vi "Heat Tapes.vi"() -> ()   [LabVIEW 2013]
panel:
  out "Boolean 7":bool
  out "Boolean 6":bool
  out "Boolean 5":bool
  out "Boolean 4":bool
  out "Boolean 3":bool
  out "Boolean 2":bool
  out "Boolean":bool
  in  "On 8":bool
  out "HT-301 Steam":dynamicdata(graph)
  in  "HT-301 SP":dbl
  in  "Auto 7":bool=TRUE
  in  "Set All":bool
  in  "Setpoint":dbl
  in  "Auto":bool
  in  "On":bool
  in  "HT-601 SP":dbl
  in  "Auto 6":bool
  in  "HT-621 SP":dbl
  in  "On 6":bool
  in  "Auto 5":bool
  in  "HT-620 SP":dbl
  in  "On 5":bool
  in  "Auto 4":bool
  in  "HT-611 SP":dbl
  in  "On 4":bool
  in  "Auto 3":bool
  in  "HT-610 SP":dbl
  in  "On 3":bool
  in  "Auto 2":bool
  in  "HT-602 SP":dbl
  in  "On 2":bool
  out "HT-601 - Ash Knockout":dynamicdata(graph)
  out "HT-602 - Horizontal":dynamicdata(graph)
  out "HT-610 - Filter 1":dynamicdata(graph)
  out "HT-620 - Filter 2":dynamicdata(graph)
  out "HT-611 - Between Filters":dynamicdata(graph)
  out "HT-621 - Between Filter 2 & VLS":dynamicdata(graph)
  in  "Auto 9":bool=TRUE
  # "Heat Tape Control Panel (to set all)"
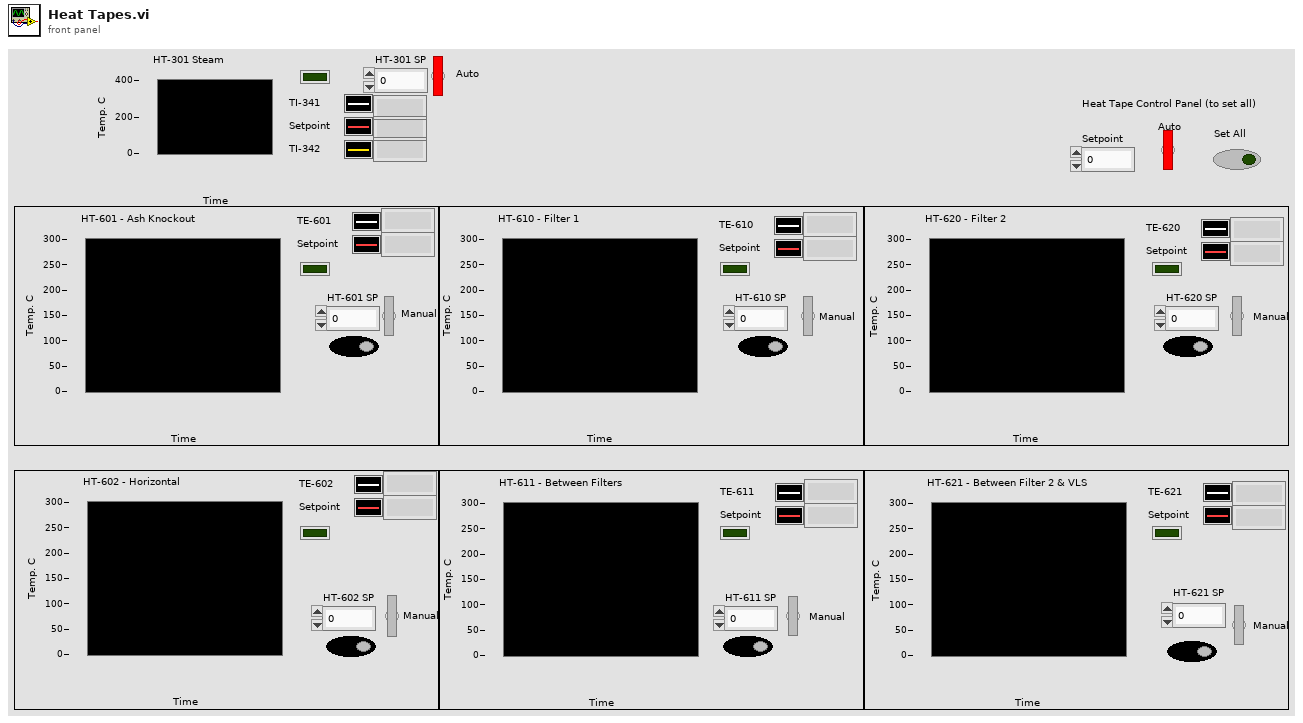
[diagram p1: front panel]
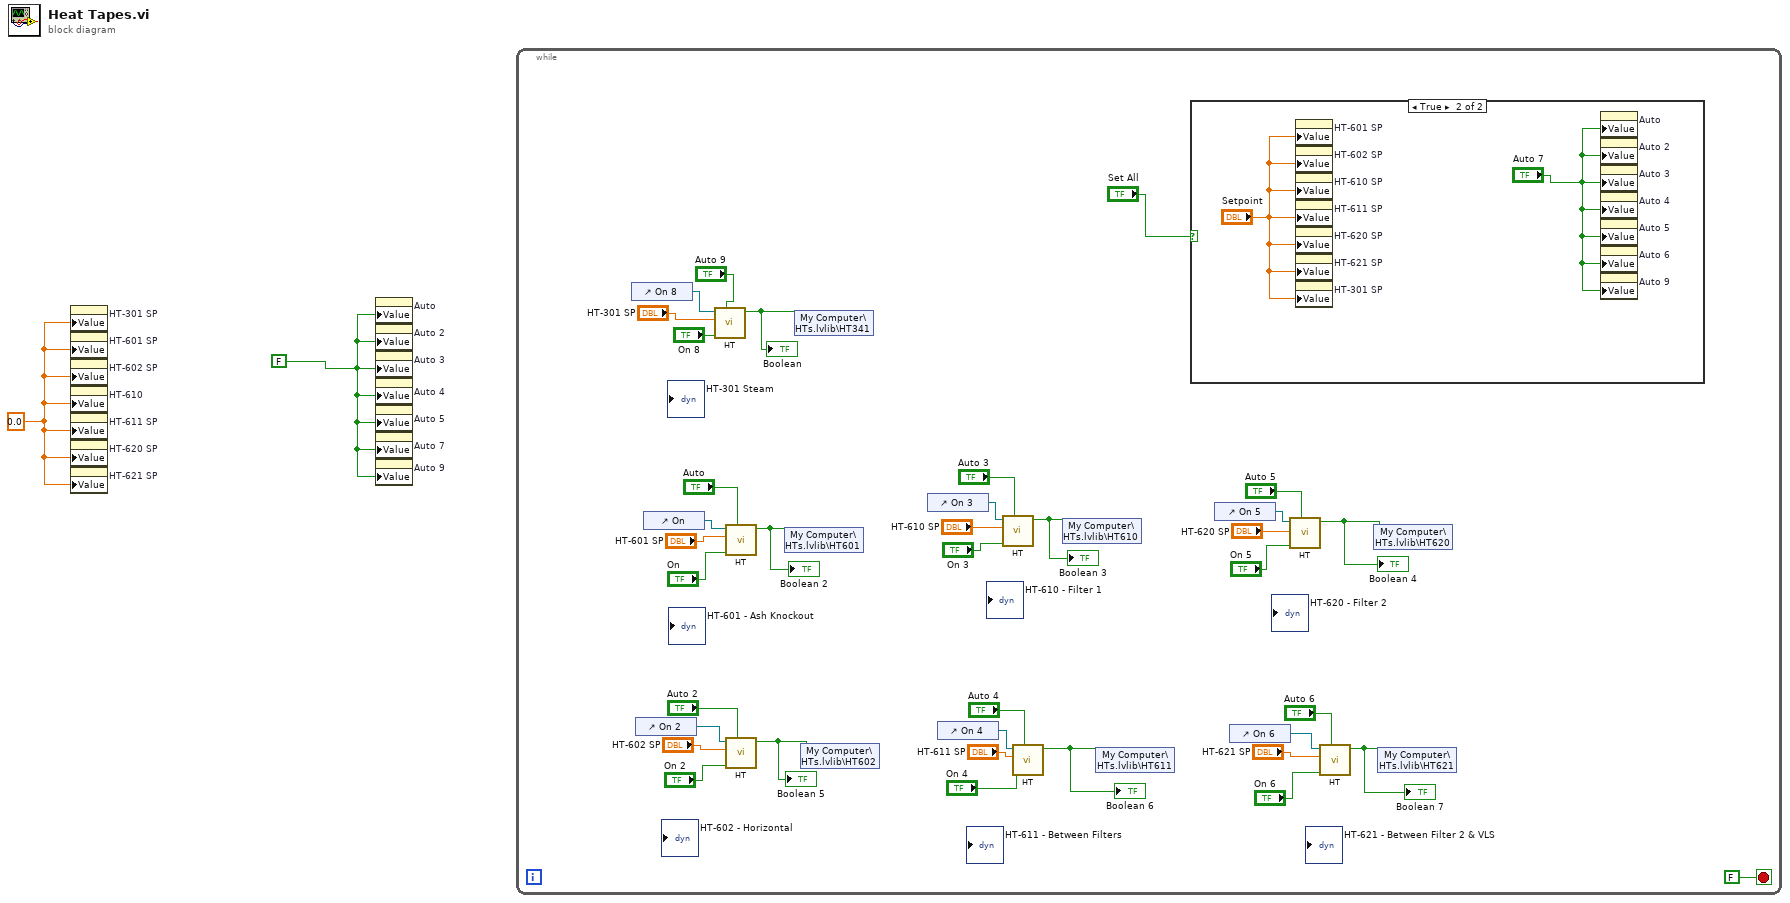
[diagram p0: block diagram]
diagram:
  w2 = FALSE ("Auto 8")
  w1 = 0.0 ("Setpoint 2")
  n1 = property on="HT-301 SP" class="DigNum (strict)"("Value"=w1) -> ()  [unwired: 2 in, 2 out]
  n2 = property on="HT-601 SP" class="DigNum (strict)"("Value"=w1) -> ()  [unwired: 2 in, 2 out]
  n3 = property on="HT-602 SP" class="DigNum (strict)"("Value"=w1) -> ()  [unwired: 2 in, 2 out]
  n4 = property on="HT-610" class="DigNum (strict)"("Value"=w1) -> ()  [unwired: 2 in, 2 out]
  n5 = property on="HT-611 SP" class="DigNum (strict)"("Value"=w1) -> ()  [unwired: 2 in, 2 out]
  n6 = property on="HT-620 SP" class="DigNum (strict)"("Value"=w1) -> ()  [unwired: 2 in, 2 out]
  n7 = property on="HT-621 SP" class="DigNum (strict)"("Value"=w1) -> ()  [unwired: 2 in, 2 out]
  n8 = property on="Auto" class="Bool (strict)"("Value"=w2) -> ()  [unwired: 2 in, 2 out]
  n9 = property on="Auto 2" class="Bool (strict)"("Value"=w2) -> ()  [unwired: 2 in, 2 out]
  n10 = property on="Auto 3" class="Bool (strict)"("Value"=w2) -> ()  [unwired: 2 in, 2 out]
  n11 = property on="Auto 4" class="Bool (strict)"("Value"=w2) -> ()  [unwired: 2 in, 2 out]
  n12 = property on="Auto 5" class="Bool (strict)"("Value"=w2) -> ()  [unwired: 2 in, 2 out]
  n13 = property on="Auto 7" class="Bool (strict)"("Value"=w2) -> ()  [unwired: 2 in, 2 out]
  n14 = property on="Auto 9" class="Bool (strict)"("Value"=w2) -> ()  [unwired: 2 in, 2 out]
  n15 = while {
    stop <- FALSE stop-if-true
    n16 = control-ref of="On 8"() -> (w12:refnum<vi>)
    n17 = control-ref of="On 2"() -> (w17:refnum<vi>)
    n18 = control-ref of="On"() -> (w16:refnum<vi>)
    n19 = call "HT.vi"("Auto"="Auto 9", "On"="On 8", "SP"="HT-301 SP", "Bool Refnum"=w12) -> ("s? t:f"=w11:bool)  [unwired: 7 in]
    "Boolean" <- w11
    n20 = call "HT.vi"("Auto"="Auto", "On"="On", "SP"="HT-601 SP", "Bool Refnum"=w16) -> ("s? t:f"=w9:bool)  [unwired: 7 in]
    "Boolean 2" <- w9
    n21 = call "HT.vi"("Auto"="Auto 2", "On"="On 2", "SP"="HT-602 SP", "Bool Refnum"=w17) -> ("s? t:f"=w6:bool)  [unwired: 7 in]
    "Boolean 5" <- w6
    n22 = shared-variable "My Computer\\HTs.lvlib\\HT601"(w9) -> ()  [unwired: 1 in, 1 out]
    n23 = shared-variable "My Computer\\HTs.lvlib\\HT341"(w11) -> ()  [unwired: 1 in, 1 out]
    n24 = shared-variable "My Computer\\HTs.lvlib\\HT602"(w6) -> ()  [unwired: 1 in, 1 out]
    n25 = control-ref of="On 3"() -> (w18:refnum<vi>)
    n26 = control-ref of="On 4"() -> (w19:refnum<vi>)
    n27 = call "HT.vi"("Auto"="Auto 3", "On"="On 3", "SP"="HT-610 SP", "Bool Refnum"=w18) -> ("s? t:f"=w8:bool)  [unwired: 7 in]
    "Boolean 3" <- w8
    n28 = call "HT.vi"("Auto"="Auto 4", "On"="On 4", "SP"="HT-611 SP", "Bool Refnum"=w19) -> ("s? t:f"=w5:bool)  [unwired: 7 in]
    "Boolean 6" <- w5
    n29 = shared-variable "My Computer\\HTs.lvlib\\HT610"(w8) -> ()  [unwired: 1 in, 1 out]
    n30 = shared-variable "My Computer\\HTs.lvlib\\HT611"(w5) -> ()  [unwired: 1 in, 1 out]
    n31 = case shown="True" "Set All" {
      frame False {
      }
      frame True {
        n32 = property on="HT-601 SP" class="DigNum (strict)"("Value"="Setpoint") -> ()  [unwired: 2 in, 2 out]
        n33 = property on="HT-602 SP" class="DigNum (strict)"("Value"="Setpoint") -> ()  [unwired: 2 in, 2 out]
        n34 = property on="HT-610 SP" class="DigNum (strict)"("Value"="Setpoint") -> ()  [unwired: 2 in, 2 out]
        n35 = property on="HT-611 SP" class="DigNum (strict)"("Value"="Setpoint") -> ()  [unwired: 2 in, 2 out]
        n36 = property on="HT-620 SP" class="DigNum (strict)"("Value"="Setpoint") -> ()  [unwired: 2 in, 2 out]
        n37 = property on="HT-621 SP" class="DigNum (strict)"("Value"="Setpoint") -> ()  [unwired: 2 in, 2 out]
        n38 = property on="HT-301 SP" class="DigNum (strict)"("Value"="Setpoint") -> ()  [unwired: 2 in, 2 out]
        n39 = property on="Auto" class="Bool (strict)"("Value"="Auto 7") -> ()  [unwired: 2 in, 2 out]
        n40 = property on="Auto 2" class="Bool (strict)"("Value"="Auto 7") -> ()  [unwired: 2 in, 2 out]
        n41 = property on="Auto 3" class="Bool (strict)"("Value"="Auto 7") -> ()  [unwired: 2 in, 2 out]
        n42 = property on="Auto 4" class="Bool (strict)"("Value"="Auto 7") -> ()  [unwired: 2 in, 2 out]
        n43 = property on="Auto 5" class="Bool (strict)"("Value"="Auto 7") -> ()  [unwired: 2 in, 2 out]
        n44 = property on="Auto 6" class="Bool (strict)"("Value"="Auto 7") -> ()  [unwired: 2 in, 2 out]
        n45 = property on="Auto 9" class="Bool (strict)"("Value"="Auto 7") -> ()  [unwired: 2 in, 2 out]
      }
    }
    n46 = control-ref of="On 5"() -> (w20:refnum<vi>)
    n47 = control-ref of="On 6"() -> (w21:refnum<vi>)
    n48 = call "HT.vi"("Auto"="Auto 5", "On"="On 5", "SP"="HT-620 SP", "Bool Refnum"=w20) -> ("s? t:f"=w7:bool)  [unwired: 7 in]
    "Boolean 4" <- w7
    n49 = call "HT.vi"("Auto"="Auto 6", "On"="On 6", "SP"="HT-621 SP", "Bool Refnum"=w21) -> ("s? t:f"=w4:bool)  [unwired: 7 in]
    "Boolean 7" <- w4
    n50 = shared-variable "My Computer\\HTs.lvlib\\HT620"(w7) -> ()  [unwired: 1 in, 1 out]
    n51 = shared-variable "My Computer\\HTs.lvlib\\HT621"(w4) -> ()  [unwired: 1 in, 1 out]
  }
